vi "Processing Loop.vi"(8 "error in":errorcluster, 11 "Broker in":refnum<class "Broker.lvclass">) -> (0 "error out":errorcluster, 3 "Broker out":refnum<class "Broker.lvclass">)   [LabVIEW 2014, in "Broker.lvclass"]
uses:
  Broker.lvclass
  Topic_class/Topic.lvclass
  Message_class/Message.lvclass
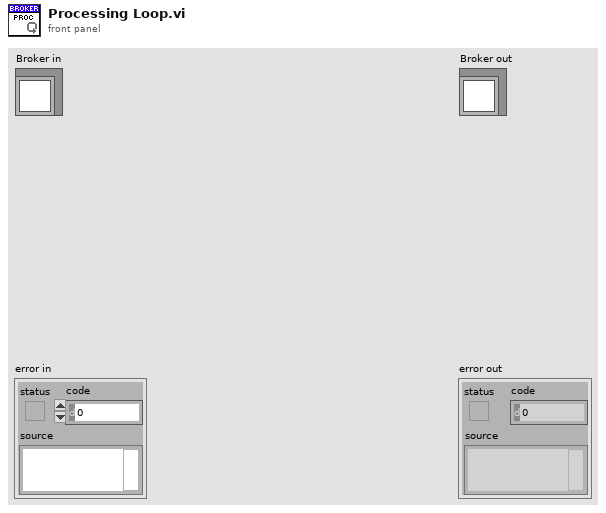
[diagram p1: front panel]
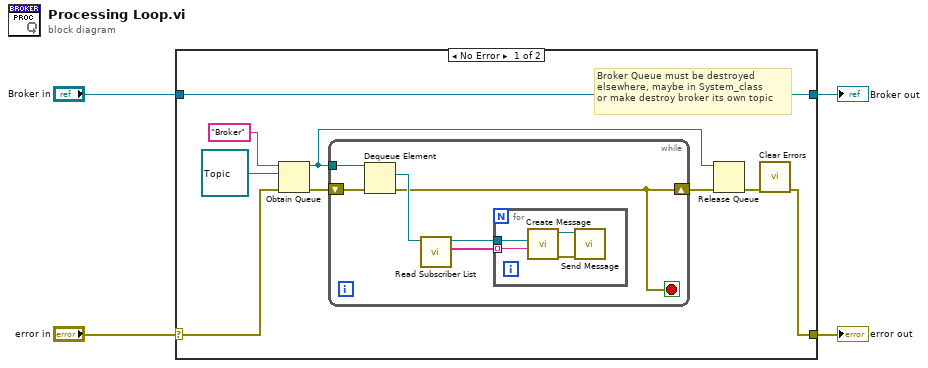
[diagram p0: block diagram]
diagram:
  n1 = case shown="No Error" "error in" {
    selector: "error in" -> [w7 w25]
    tunnel: [w5 w25] -> w3
    tunnel: [w13 w24] -> w1
    tunnel: "Broker in" -> [w13 w24]
    frame No Error {
      # "Broker Queue must be destroyed\nelsewhere, maybe in System_class\nor make destroy broker its own topic"
      n2 = Obtain Queue(name (unnamed)="Broker", element data type=refnum<class "Topic.lvclass"> refnum ("Topic.lvclass"), error in (no error)=w7) -> (queue out=w8:refnum<queue>, error out=w10:errorcluster)  [unwired: 2 in, 1 out]
      n3 = while {
        tunnel: w8 -> [w19]
        shift-right: [w14] -> w9
        shift-left: w10 -> [w18]
        stop <- w14 stop-if-true
        n4 = Dequeue Element(queue=w19, error in (no error)=w18) -> (element=w17:refnum<class "Topic.lvclass">, error out=w14:errorcluster)  [unwired: 1 in, 2 out]
        n5 = call-dynamic "Read Subscriber List.vi"("Topic in"=w17) -> ("Subscriber List"=w16:string[], "Topic out"=w15:refnum<class "Topic.lvclass">)  [unwired: 8 in, 1 out]
        n6 = for {
          tunnel: w16 -> [w21] mode=indexing
          tunnel: w15 -> [w20]
          n7 = call-dynamic "Create Message.vi"("Client ID"=w21, "Topic.lvclass"=w20) -> ("error out"=w23:errorcluster, "Message out"=w22:refnum<class "Message.lvclass">)  [unwired: 8 in]
          n8 = call-dynamic "Send Message.vi"("error in"=w23, "Message in"=w22) -> ()  [unwired: 8 in, 2 out]
        }
      }
      n9 = Release Queue(queue=w8, error in (no error)=w9) -> (error out=w6:errorcluster)  [unwired: 1 in, 2 out]
      n10 = call <vilib>:"Clear Errors.vi"("error in (no error)"=w6) -> ("error out"=w5:errorcluster)  [unwired: 5 in, 1 out]
    }
    frame Error {
    }
  }
  "error out" <- w3
  "Broker out" <- w1
